vi "Finish Update.vi"(8 "instVIref":T1, 11 "FPGAtarget in":refnum<class "FPGATarget.lvclass">) -> (3 "FPGAtarget out":refnum<class "FPGATarget.lvclass">)   [LabVIEW 2020, in "NI_TargetHelper.lvlib" / "FPGATarget.lvclass"]
uses:
  <vilib>/TargetSupport/NI_TargetHelper/FPGATarget/FPGATarget.lvclass
  <vilib>/TargetSupport/NI_TargetHelper/Instance VIref.ctl
  <vilib>/Utility/miscctls.llb/LVPointTypeDef.ctl
  <vilib>/TargetSupport/NI_TargetHelper/FPGATarget/FPGATarget.lvclass/FPGATarget.ctl
  <vilib>/TargetSupport/NI_TargetHelper/NI_TargetHelper.lvlib
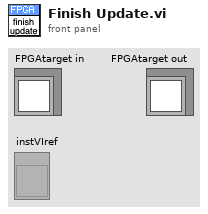
[diagram p1: front panel]
types:
  T1 = typedef "NI_TargetHelper.lvlib/Instance VIref.ctl" = refnum<vi>
  T2 = typedef "LVPointTypeDef.ctl" = cluster{"Horizontal":i16, "Vertical":i16}
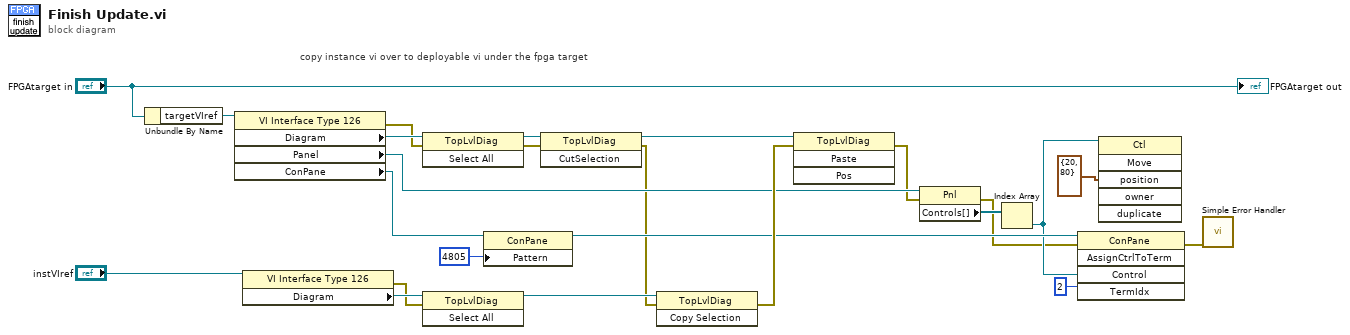
[diagram p0: block diagram]
diagram:
  # "copy instance vi over to deployable vi under the fpga target"
  n1 = Unbundle By Name("FPGAtarget in") -> ("targetVIref"=w24:T1)
  n2 = property class="VI Interface Type 126"(reference=w24) -> (error out=w7:errorcluster, "Diagram"=w23:refnum<vi>, "Panel"=w13:refnum<vi>, "ConPane"=w16:refnum<vi>)  [unwired: 1 in, 1 out]
  n3 = property class="VI Interface Type 126"(reference="instVIref") -> (error out=w8:errorcluster, "Diagram"=w20:refnum<vi>)  [unwired: 1 in, 1 out]
  n4 = invoke class="TopLvlDiag" method="Select All"(reference=w23, error in=w7) -> (reference out=w22:refnum<vi>, error out=w6:errorcluster)  [unwired: 1 in, 1 out]
  n5 = invoke class="TopLvlDiag" method="Select All"(reference=w20, error in=w8) -> (reference out=w21:refnum<vi>)  [unwired: 1 in, 2 out]
  n6 = property class="ConPane"(reference=w16, "Pattern"=u32 4805) -> (reference out=w14:refnum<vi>)  [unwired: 1 in, 1 out]
  n7 = invoke class="TopLvlDiag" method="CutSelection"(reference=w22, error in=w6) -> (reference out=w19:refnum<vi>, error out=w3:errorcluster)  [unwired: 1 in, 1 out]
  n8 = invoke class="TopLvlDiag" method="Copy Selection"(reference=w21, error in=w3) -> (error out=w18:errorcluster)  [unwired: 1 in, 2 out]
  n9 = invoke class="TopLvlDiag" method="Paste"(reference=w19, error in=w18) -> (error out=w11:errorcluster)  [unwired: 2 in, 3 out]
  n10 = property class="Pnl"(reference=w13, error in=w11) -> (error out=w5:errorcluster, "Controls[]"=w12:refnum<vi>[])  [unwired: 1 out]
  n11 = Index Array(array=w12) -> (element=w10:refnum<vi>)  [unwired: 1 in]
  n12 = invoke class="ConPane" method="AssignCtrlToTerm"(reference=w14, error in=w5, "Control"=w10, "TermIdx"=u32 2 ("Terminal Index")) -> (error out=w4:errorcluster)  [unwired: 1 in, 4 out]
  n13 = invoke class="Ctl" method="Move"(reference=w10, "position"=T2 {"Horizontal"=20, "Vertical"=80} ("location")) -> ()  [unwired: 4 in, 6 out]
  n14 = call <vilib>:"Simple Error Handler.vi"("error in (no error)"=w4) -> ()  [unwired: 4 in, 5 out]
  "FPGAtarget out" <- "FPGAtarget in"
